vi "DAQmx.Read Buffer Params.vi"(8 "error in (no error)":errorcluster, 11 "DAQmx in":refnum<class "DAQmx.lvclass">) -> (0 "error out":errorcluster, 3 "DAQmx out":refnum<class "DAQmx.lvclass">)   [LabVIEW 2019, in "DAQmx.lvclass"]
uses:
  DAQmx.lvclass
  DAQmx.lvclass/DAQmx.ctl
  <resource>/objmgr/daqmx.rc
panel:
  out "AI DataXfer":i32[](array[ring]) items=["Onboard Memory More than Half Full"=10237, "Onboard Memory Not Empty"=10241, "Onboard Memory Custom Threshold"=12577, "When Acquisition Complete"=12546]
  out "AO DataXfer":i32[](array[ring]) items=["Onboard Memory Empty"=10235, "Onboard Memory Half Full or Less"=10239, "Onboard Memory Less than Full"=10242]
  out "Fs (S/s)":dbl=204800.0000286 format="%#_13g"
  out "Timebase (Hz)":dbl=204800.0000286 format="%#_13g"
  out "Output.Onboard Buffer":u32[](array[numeric])
  out "Output.Buffer":u32[](array[numeric])
  out "Input.Onboard Buffer":u32[](array[numeric])
  out "Input.Buffer":u32[](array[numeric])
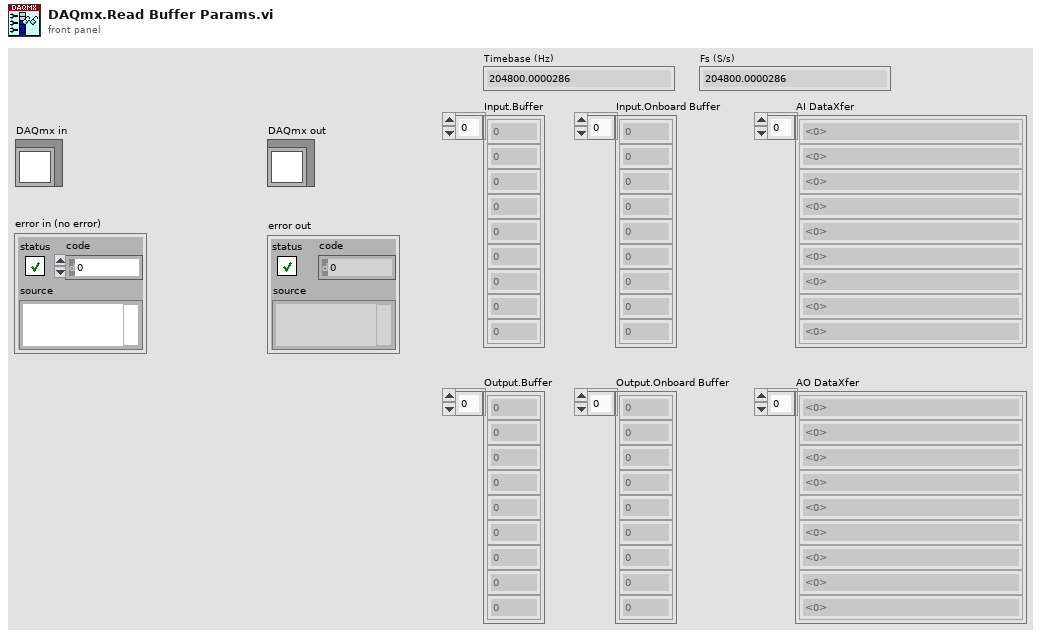
[diagram p1: front panel]
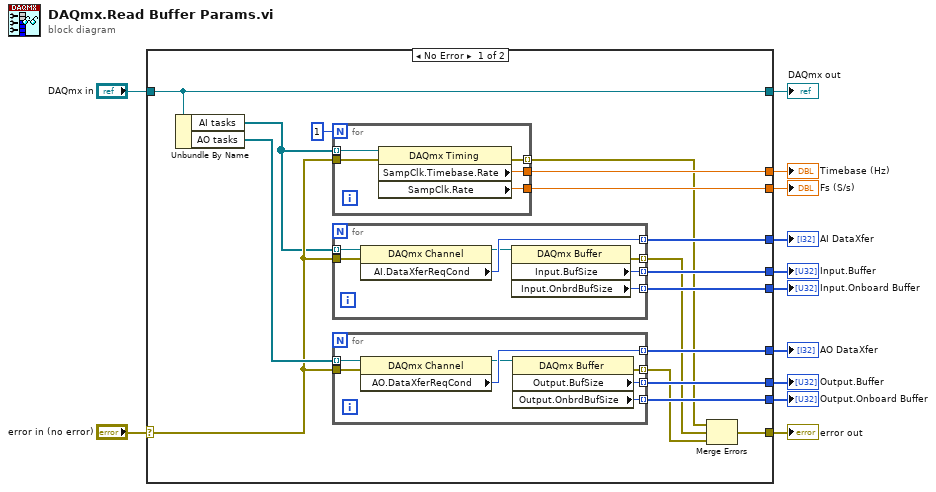
[diagram p0: block diagram]
diagram:
  n1 = case shown="No Error" "error in (no error)" {
    selector: "error in (no error)" -> [w16 w50]
    tunnel: [w15 w50] -> w12
    tunnel: [w20 w49] -> w10
    tunnel: "DAQmx in" -> [w20 w49]
    tunnel: [w28 _] -> w8
    tunnel: [w27 _] -> w7
    tunnel: [w26 _] -> w6
    tunnel: [w25 _] -> w5
    tunnel: [w24 _] -> w4
    tunnel: [w23 _] -> w3
    tunnel: [w22 _] -> w2
    tunnel: [w21 _] -> w1
    frame No Error {
      n2 = Unbundle By Name(w20) -> ("AI tasks"=w14:refnum<k21>[], "AO tasks"=w29:refnum<k21>[])
      n3 = for {
        N: 1 -> [_]
        tunnel: w14 -> [w34] mode=indexing
        tunnel: w16 -> [w33]
        tunnel: [w32] -> w25
        tunnel: [w31] -> w26
        tunnel: [w30] -> w19 mode=indexing
        n4 = property class="DAQmx Timing"(reference=w34, error in=w33) -> (error out=w30:errorcluster, "SampClk.Timebase.Rate"=w32:dbl, "SampClk.Rate"=w31:dbl)  [unwired: 1 out]
      }
      n5 = for {
        tunnel: w14 -> [w44] mode=indexing
        tunnel: [w48] -> w21 mode=indexing
        tunnel: [w47] -> w22 mode=indexing
        tunnel: w16 -> [w43]
        tunnel: [w46] -> w28 mode=indexing
        tunnel: [w42] -> w18 mode=indexing
        n6 = property class="DAQmx Channel"(reference=w44, error in=w43) -> (reference out=w45:refnum<k21>, "AI.DataXferReqCond"=w46:i32)  [unwired: 1 out]
        n7 = property class="DAQmx Buffer"(reference=w45) -> (error out=w42:errorcluster, "Input.BufSize"=w48:u32, "Input.OnbrdBufSize"=w47:u32)  [unwired: 1 in, 1 out]
      }
      n8 = for {
        tunnel: w29 -> [w38] mode=indexing
        tunnel: [w41] -> w23 mode=indexing
        tunnel: [w40] -> w24 mode=indexing
        tunnel: w16 -> [w36]
        tunnel: [w39] -> w27 mode=indexing
        tunnel: [w35] -> w17 mode=indexing
        n9 = property class="DAQmx Channel"(reference=w38, error in=w36) -> (reference out=w37:refnum<k21>, "AO.DataXferReqCond"=w39:i32)  [unwired: 1 out]
        n10 = property class="DAQmx Buffer"(reference=w37) -> (error out=w35:errorcluster, "Output.BufSize"=w41:u32, "Output.OnbrdBufSize"=w40:u32)  [unwired: 1 in, 1 out]
      }
      n11 = Merge Errors(w19, w18, w17) -> (w15:errorcluster)
    }
    frame Error {
    }
  }
  "error out" <- w12
  "DAQmx out" <- w10
  "Input.Buffer" <- w1
  "Input.Onboard Buffer" <- w2
  "Output.Buffer" <- w3
  "Output.Onboard Buffer" <- w4
  "Timebase (Hz)" <- w5
  "Fs (S/s)" <- w6
  "AO DataXfer" <- w7
  "AI DataXfer" <- w8
